vi "LoadAndRun.vi"(3 "error in (no error)":errorcluster caption="错误输入（无错误）", 4 "run?":bool caption="运行？", 5 "path":path caption="路径") -> (0 "error out":errorcluster caption="错误输出", 2 "vi refnum out":refnum<vi> caption="VI引用句柄输出")   [LabVIEW 2013]
doc: "打开一个指定VI的引用句柄，运行VI。"
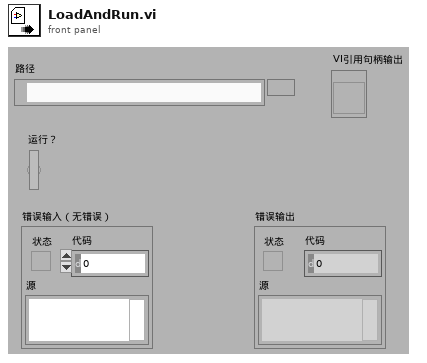
[diagram p1: front panel]
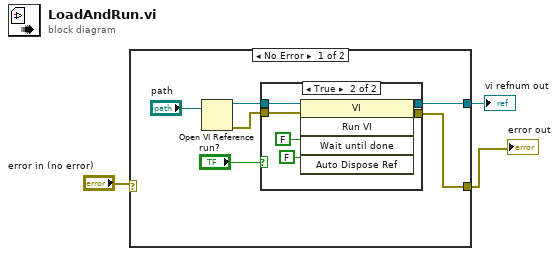
[diagram p0: block diagram]
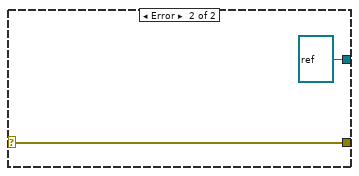
[diagram p3: hidden frame]
diagram:
  n1 = case shown="No Error" "error in (no error)" {
    selector: "error in (no error)" -> [_ w18]
    tunnel: [w6 refnum<vi> refnum] -> w2
    tunnel: [w4 w18] -> w1
    frame No Error {
      n2 = Open VI Reference(vi path="path") -> (vi reference=w7:refnum<vi>, error out=w5:errorcluster)  [unwired: 5 in]
      n3 = case shown="True" "run?" {
        tunnel: w7 -> [w11 w17]
        tunnel: [w11 w15] -> w6
        tunnel: w5 -> [w10 w14]
        tunnel: [w10 w13] -> w4
        frame False {
        }
        frame True {
          n4 = invoke class="VI" method="Run VI"(reference=w17, error in=w14, "Wait until done"=FALSE, "Auto Dispose Ref"=FALSE ("自动销毁引用")) -> (reference out=w15:refnum<vi>, error out=w13:errorcluster)  [unwired: 1 in, 3 out]
        }
      }
    }
    frame Error {
    }
  }
  "vi refnum out" <- w2
  "error out" <- w1
